vi "TBM HDI Wirebonds.vi"(6 "Match Offset (Pattern Matching 1)":cluster{"X":sgl, "Y":sgl}, 8 "Minimum Match Score (Pattern Matching 1)":sgl=600.0, 9 "controller in":refnum<k24>, 10 "Template for Encapsulation pattern matching":path, 11 "T/B/L/R":i32) -> (0 "error out":errorcluster, 1 "Number of Matches (Pattern Matching 1)":i32, 3 "Match(es) Found":bool)   [LabVIEW 2011]
uses:
  C:/Users/Admin/Desktop/Gantry Code Transfer/source/Code Transfer/Aerotech.A3200.dll
  Aerotech.A3200.dll
  Template change for pattern match.vi
  <vilib>/vision/driver/NI_Vision_Acquisition_Software.lvlib
  <vilib>/vision/NI_Vision_Development_Module.lvlib
panel:
  in  "Scale Factor":sgl=0.000429
  out "y rel move":dbl
  out "x rel move":dbl
  out "y":sgl
  out "x":sgl
  out "Image Out":T1(plugin-control)
  out "Calibrated Matches":T2(array[cluster]) {"Bounding Box"."y" format="%.2f"; "Bounding Box"."x" format="%.2f"; "Position"."y" format="%.2f"; "Position"."x" format="%.2f"; "Score" format="%.2f"; "Scale" format="%.2f"; "Angle" format="%.2f"}
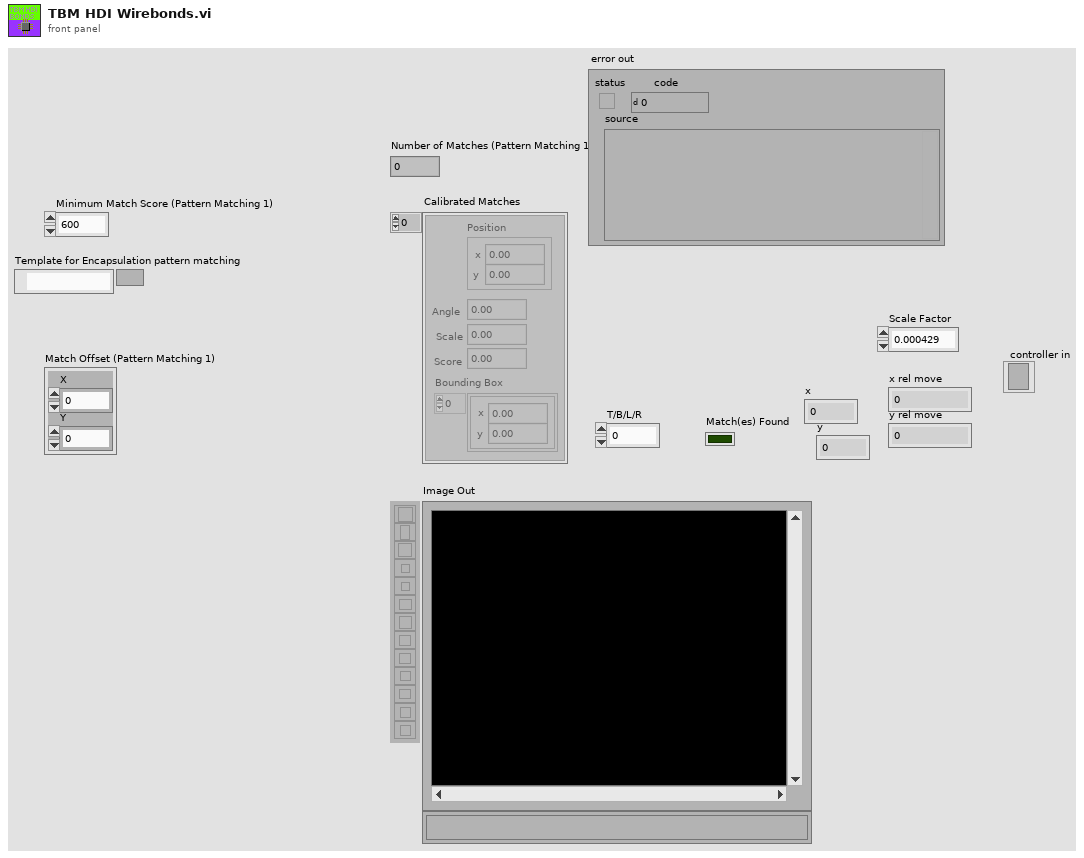
[diagram p1: front panel]
types:
  T1 = typedef "IMAQ Image.ctl" = refnum<image>
  T2 = cluster{"Position":cluster{"x":sgl, "y":sgl}, "Angle":sgl, "Scale":sgl, "Score":sgl, "Bounding Box":cluster{"x":sgl, "y":sgl}[]}[]
  T3 = cluster{"Global Rectangle":i32[], "Contours":cluster{"ID":enum32{"External", "Internal"}, "Type":u32, "Coordinates":i32[]}[]}
  T4 = typedef "IMAQdx.ctl" = refnum<k21>
  T5 = cluster{"Match Mode":u16, "Subpixel Accuracy":bool, "Rotation Angle Ranges (degrees) (Pattern Matching 1)":cluster{sgl, sgl}[]}
  T6 = cluster{"Global Rectangle":i32[], "Number of Matches Requested (Pattern Matching 1)":i32, "Minimum Match Score (Pattern Matching 1)":sgl}
  T7 = cluster{"Position":cluster{"x":sgl, "y":sgl}, "Angle":sgl, "Scale":sgl, "Score":sgl, "Bounding Box":cluster{"x":sgl, "y":sgl}[]}
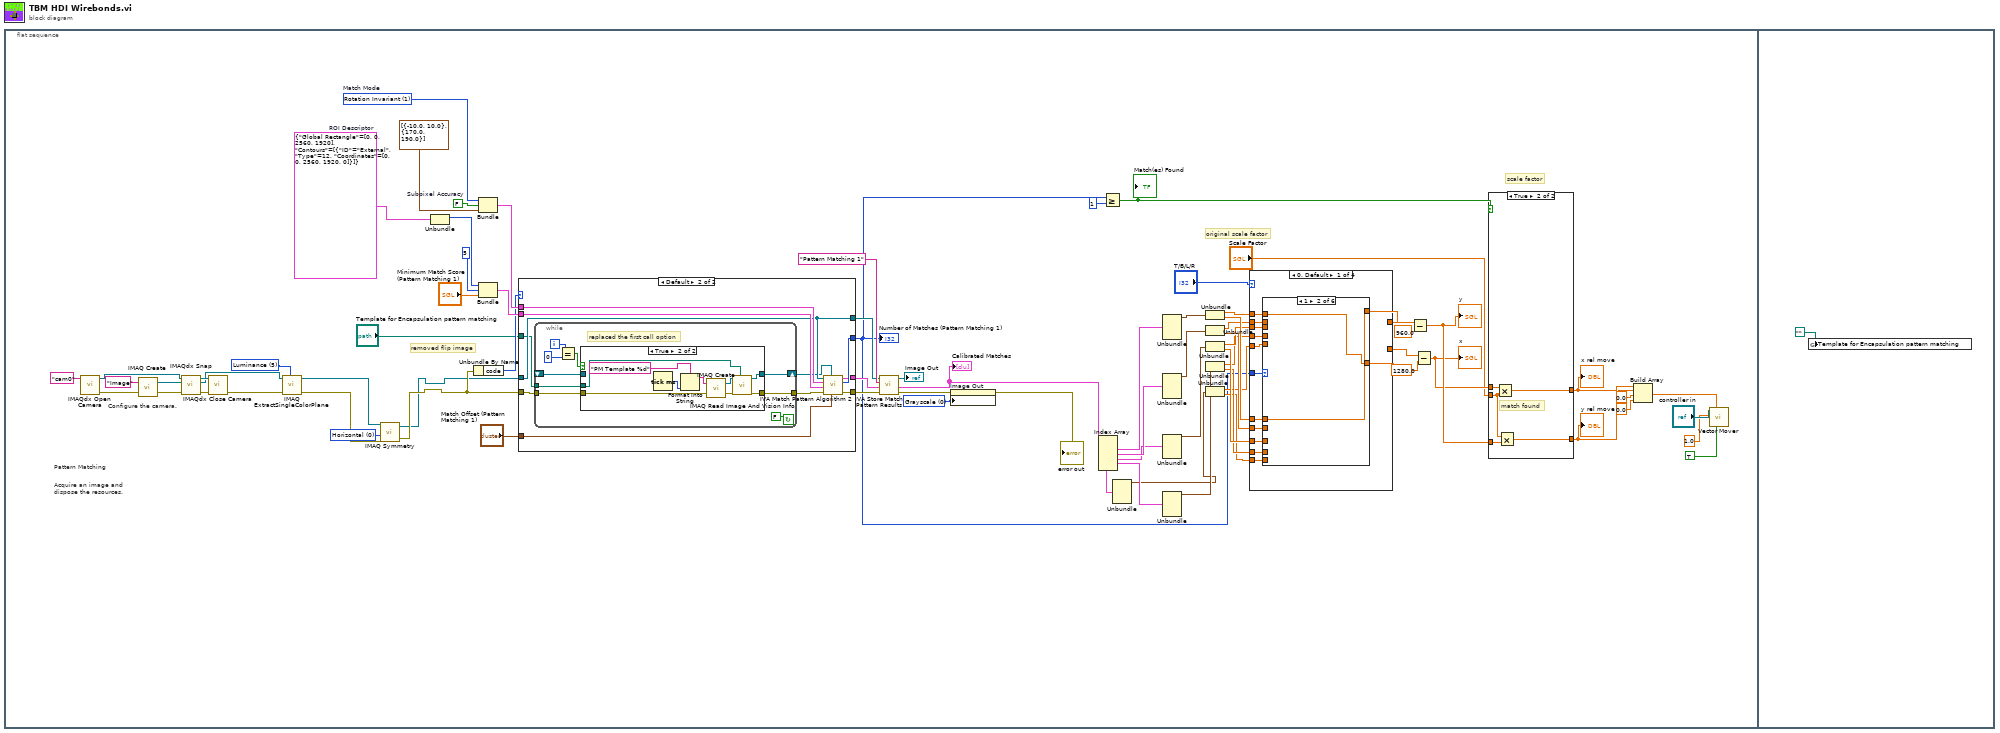
[diagram p0: block diagram]
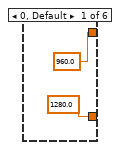
[diagram p2: hidden frame]
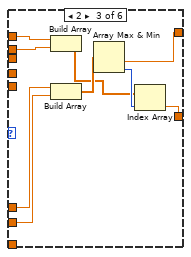
[diagram p3: hidden frame]
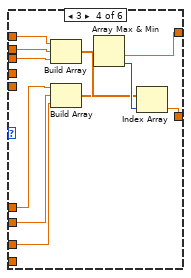
[diagram p4: hidden frame]
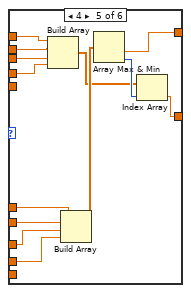
[diagram p5: hidden frame]
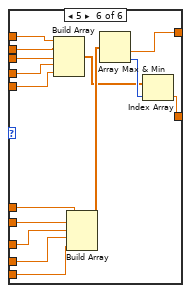
[diagram p6: hidden frame]
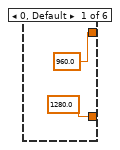
[diagram p8: hidden frame]
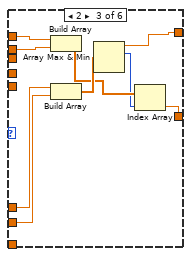
[diagram p9: hidden frame]
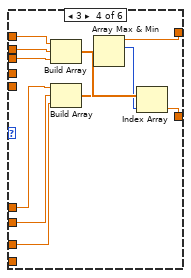
[diagram p10: hidden frame]
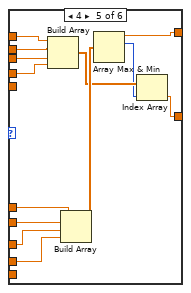
[diagram p11: hidden frame]
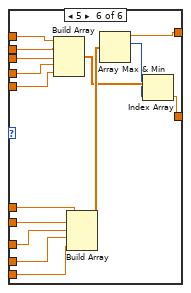
[diagram p12: hidden frame]
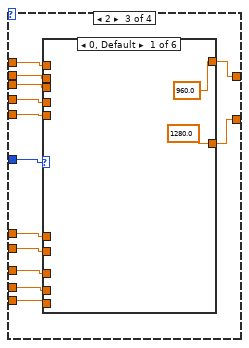
[diagram p13: hidden frame]
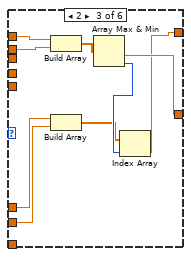
[diagram p15: hidden frame]
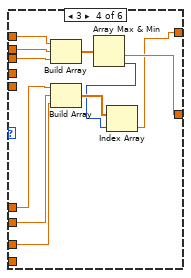
[diagram p16: hidden frame]
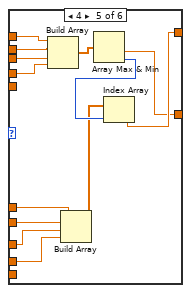
[diagram p17: hidden frame]
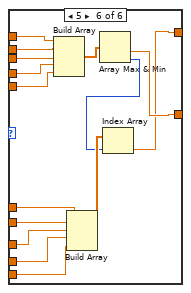
[diagram p18: hidden frame]
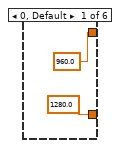
[diagram p20: hidden frame]
diagram:
  n1 = flat-sequence {
    frame #0 {
      w5 = u32 0 items=["Horizontal", "Vertical", "Central", "1st Diagonal", "2nd Diagonal"] ("Type of Symmetry")
      w47 = u32 0 items=["Grayscale", "Binary", "Gradient", "Rainbow", "Temperature", "User Defined"] ("Palette")
      w63 = FALSE  # Subpixel Accuracy
      w64 = u16 1 items=["Shift Invariant", "Rotation Invariant"]  # Match Mode
      w53 = T3 {"Global Rectangle"=[0, 0, 2560, 1920], "Contours"=[{"ID"=enum."External", "Type"=12, "Coordinates"=[0, 0, 2560, 1920, 0]}]}  # ROI Descriptor
      w66 = 5 items=["Red", "Green", "Blue", "Hue", "Saturation", "Luminance", "Value", "Intensity"] ("Color Plane")
      # "removed flip image"
      # "original scale factor"
      # "scale factor"
      # "Pattern Matching"
      # "Acquire an image and\ndispose the resources."
      # "Configure the camera."
      n2 = call <vilib>:"IMAQdx Open Camera.vi"("Session In"="cam0" ("Interface Name")) -> ("error out"=w73:errorcluster, "Session Out"=w67:T4)  [unwired: 9 in]
      n3 = call "IMAQ Create"("Image Name"="Image", "error in (no error)"=w73) -> ("New Image"=w69:T1, "error out"=w68:errorcluster)  [unwired: 3 in]
      n4 = call <vilib>:"IMAQdx Snap.vi"("error in"=w68, "Image In"=w69, "Session In"=w67) -> ("error out"=w71:errorcluster, "Image Out"=w65:T1, "Session Out"=w72:T4)  [unwired: 6 in]
      n5 = call <vilib>:"IMAQdx Close Camera.vi"("error in"=w71, "Session In"=w72) -> ("error out"=w70:errorcluster)  [unwired: 9 in]
      n6 = call "IMAQ ExtractSingleColorPlane"("Color Plane"=w66, "error in (no error)"=w70, "Image Src"=w65) -> ("error out"=w3:errorcluster, "Image Dst Out"=w4:T1)  [unwired: 7 in]
      n7 = call "IMAQ Symmetry"("error in (no error)"=w3, "Type of Symmetry"=w5, "Image Src"=w4) -> ("error out"=w2:errorcluster, "Image Dst Out"=w1:T1)  [unwired: 2 in]
      n8 = Unbundle(w53) -> ("Global Rectangle"=w52:i32[])  [unwired: 1 out]
      n9 = Unbundle By Name(w2) -> ("code"=w49:i32)
      n10 = Bundle("Match Mode"=w64, "Subpixel Accuracy"=w63, "Rotation Angle Ranges (degrees) (Pattern Matching 1)"=cluster{sgl, sgl}[] [{-10.0, 10.0}, {170.0, 190.0}]) -> (w61:T5)  [unwired: 1 in]
      n11 = Bundle("Global Rectangle"=w52, "Number of Matches Requested (Pattern Matching 1)"=5, "Minimum Match Score (Pattern Matching 1)"="Minimum Match Score (Pattern Matching 1)") -> (w58:T6)  [unwired: 1 in]
      n12 = case shown="Default" w49 {
        tunnel: "Template for Encapsulation pattern matching" -> [_ w346]
        tunnel: w2 -> [_ w345]
        tunnel: [_ w353] -> w7
        tunnel: w61 -> [_ w352]
        tunnel: w58 -> [_ w351]
        tunnel: "Match Offset (Pattern Matching 1)" -> [_ w350]
        tunnel: w1 -> [w342 w347]
        tunnel: [_ w349] -> w55
        tunnel: [_ w348] -> w51
        tunnel: [w342 w347] -> w50
        frame -1074396199, -1074396198 {
          # "Discard\nCoordinate\nSystem Error"
        }
        frame Default {
          n13 = while {
            shift-right: [w362] -> w343
            shift-left: _ -> [w361]
            tunnel: [w359] -> w344
            tunnel: w345 -> [w358]
            tunnel: w346 -> [w357]
            i -> [w356]
            stop <- FALSE continue-if-true
            # "replaced the first call option"
            n14 = Equal?(x=w356, y=0) -> (x = y?=w354:bool)
            n15 = case shown="True" w354 {
              tunnel: [w364 w370] -> w362
              tunnel: w361 -> [w364 _]
              tunnel: [w363 w367] -> w359
              tunnel: w358 -> [w363 w366]
              tunnel: w357 -> [_ w365]
              frame False {
              }
              frame True {
                n16 = Tick Count (ms)() -> (millisecond timer value=w373:u32)
                n17 = Format Into String(format string="PM Template %d" ("Image Name"), w373) -> (resulting string=w372:string)  [unwired: 2 in, 1 out]
                n18 = call "IMAQ Create"("Image Name"=w372, "error in (no error)"=w366) -> ("New Image"=w369:T1, "error out"=w368:errorcluster)  [unwired: 3 in]
                n19 = call "IMAQ Read Image And Vision Info"("File Path"=w365, "error in (no error)"=w368, "Image"=w369) -> ("error out"=w367:errorcluster, "Image Out"=w370:T1)  [unwired: 6 in, 1 out]
              }
            }
          }
          n20 = call <vilib>:"IVA Match Pattern Algorithm 2.vi"("Match Offset"=w350, "Image Template"=w343, "error in (no error)"=w344, "Match Parameters"=w351, "Setup Match Parameters"=w352, "Image"=w347) -> ("error out"=w349:errorcluster, "Number of Matches"=w353:i32, "Matches"=w348:T2)  [unwired: 3 in]
        }
      }
      "Number of Matches (Pattern Matching 1)" <- w7
      n21 = call <vilib>:"IVA Store Match Pattern Results.vi"("error in (no error)"=w55, "Matches"=w51, "Step Name"="Pattern Matching 1", "Image in"=w50) -> ("error out"=w54:errorcluster, "Calibrated Matches"=w8:T2, "Image dup"=→"Image Out":T1)  [unwired: 5 in]
      "Calibrated Matches" <- w8
      "error out" <- w54
      n22 = property on="Image Out" class="ImageControl"(error in=w54, "Palette:Palette Type"=w47) -> ()  [unwired: 1 in, 2 out]
      n23 = Index Array(array=w8) -> (element #1=w43:T7, element #2=w42:T7, element #3=w41:T7, element #4=w40:T7, element #5=w20:T7)  [unwired: 5 in]
      n24 = Greater Or Equal?(x=w7, y=1) -> (x >= y?=w33:bool)
      "Match(es) Found" <- w33
      n25 = Unbundle(w20) -> ("Position"=w19:cluster{"x":sgl, "y":sgl})  [unwired: 4 out]
      n26 = Unbundle(w43) -> ("Position"=w36:cluster{"x":sgl, "y":sgl})  [unwired: 4 out]
      n27 = Unbundle(w42) -> ("Position"=w37:cluster{"x":sgl, "y":sgl})  [unwired: 4 out]
      n28 = Unbundle(w41) -> ("Position"=w38:cluster{"x":sgl, "y":sgl})  [unwired: 4 out]
      n29 = Unbundle(w40) -> ("Position"=w39:cluster{"x":sgl, "y":sgl})  [unwired: 4 out]
      n30 = Unbundle(w36) -> ("x"=w30:sgl, "y"=w29:sgl)
      n31 = Unbundle(w37) -> ("x"=w28:sgl, "y"=w27:sgl)
      n32 = Unbundle(w38) -> ("x"=w25:sgl, "y"=w24:sgl)
      n33 = Unbundle(w39) -> ("x"=w21:sgl, "y"=w23:sgl)
      n34 = Unbundle(w19) -> ("x"=w18:sgl, "y"=w17:sgl)
      n35 = case shown="0, Default" "T/B/L/R" {
        tunnel: w30 -> [w88 w153 w218 w283]
        tunnel: w29 -> [w87 w148 w213 w278]
        tunnel: w28 -> [w86 w152 w217 w282]
        tunnel: w27 -> [w85 w147 w212 w277]
        tunnel: [w84 w141 w206 w271] -> w26
        tunnel: w25 -> [w83 w151 w216 w281]
        tunnel: w24 -> [w82 w146 w211 w276]
        tunnel: w23 -> [w81 w145 w210 w275]
        tunnel: [w80 w142 w207 w272] -> w22
        tunnel: w21 -> [w79 w150 w215 w280]
        tunnel: w18 -> [w78 w149 w214 w279]
        tunnel: w17 -> [w77 w144 w209 w274]
        tunnel: w7 -> [w76 w143 w208 w273]
        frame 0, Default {
          n36 = case shown="1" w76 {
            tunnel: w88 -> [_ w91 w101 w109 w122 w137]
            tunnel: w87 -> [_ w92 w99 w106 w118 w133]
            tunnel: [sgl 960.0 ("y") w92 w96 w111 w124 w139] -> w84
            tunnel: w86 -> [_ _ w100 w108 w121 w136]
            tunnel: w85 -> [_ _ w98 w105 w117 w132]
            tunnel: w83 -> [_ _ _ w107 w120 w135]
            tunnel: w82 -> [_ _ _ w104 w116 w131]
            tunnel: w81 -> [_ _ _ _ w115 w130]
            tunnel: [sgl 1280.0 ("x") w91 w93 w110 w123 w138] -> w80
            tunnel: w79 -> [_ _ _ _ w119 w134]
            tunnel: w78 -> [_ _ _ _ _ w127]
            tunnel: w77 -> [_ _ _ _ _ w126]
            frame 0, Default {
            }
            frame 1 {
            }
            frame 2 {
              n37 = Build Array(w101, w100) -> (w94:sgl[])
              n38 = Build Array(w99, w98) -> (w95:sgl[])
              n39 = Array Max & Min(array=w95) -> (min value=w96:sgl, min index (indices)=w97:i32)  [unwired: 2 out]
              n40 = Index Array(array=w94, index=w97) -> (element=w93:sgl)
            }
            frame 3 {
              n41 = Build Array(w109, w108, w107) -> (w103:sgl[])
              n42 = Build Array(w106, w105, w104) -> (w102:sgl[])
              n43 = Array Max & Min(array=w102) -> (min value=w111:sgl, min index (indices)=w112:i32)  [unwired: 2 out]
              n44 = Index Array(array=w103, index=w112) -> (element=w110:sgl)
            }
            frame 4 {
              n45 = Build Array(w122, w121, w120, w119) -> (w113:sgl[])
              n46 = Build Array(w118, w117, w116, w115) -> (w114:sgl[])
              n47 = Array Max & Min(array=w114) -> (min value=w124:sgl, min index (indices)=w125:i32)  [unwired: 2 out]
              n48 = Index Array(array=w113, index=w125) -> (element=w123:sgl)
            }
            frame 5 {
              n49 = Build Array(w137, w136, w135, w134, w127) -> (w128:sgl[])
              n50 = Build Array(w133, w132, w131, w130, w126) -> (w129:sgl[])
              n51 = Array Max & Min(array=w129) -> (min value=w139:sgl, min index (indices)=w140:i32)  [unwired: 2 out]
              n52 = Index Array(array=w128, index=w140) -> (element=w138:sgl)
            }
          }
        }
        frame 1 {
          n53 = case shown="1" w143 {
            tunnel: w153 -> [_ w156 w166 w176 w189 w204]
            tunnel: w148 -> [_ w157 w164 w173 w185 w200]
            tunnel: [sgl 960.0 ("y") w157 w158 w167 w178 w192] -> w141
            tunnel: w152 -> [_ _ w165 w175 w188 w203]
            tunnel: w147 -> [_ _ w163 w172 w184 w199]
            tunnel: w151 -> [_ _ _ w174 w187 w202]
            tunnel: w146 -> [_ _ _ w171 w183 w198]
            tunnel: w145 -> [_ _ _ _ w182 w197]
            tunnel: [sgl 1280.0 ("x") w156 w160 w177 w190 w205] -> w142
            tunnel: w150 -> [_ _ _ _ w186 w201]
            tunnel: w149 -> [_ _ _ _ _ w194]
            tunnel: w144 -> [_ _ _ _ _ w193]
            frame 0, Default {
            }
            frame 1 {
            }
            frame 2 {
              n54 = Build Array(w166, w165) -> (w161:sgl[])
              n55 = Build Array(w164, w163) -> (w162:sgl[])
              n56 = Array Max & Min(array=w162) -> (max value=w158:sgl, max index (indices)=w159:i32)  [unwired: 2 out]
              n57 = Index Array(array=w161, index=w159) -> (element=w160:sgl)
            }
            frame 3 {
              n58 = Build Array(w176, w175, w174) -> (w170:sgl[])
              n59 = Build Array(w173, w172, w171) -> (w169:sgl[])
              n60 = Array Max & Min(array=w169) -> (max value=w167:sgl, max index (indices)=w168:i32)  [unwired: 2 out]
              n61 = Index Array(array=w170, index=w168) -> (element=w177:sgl)
            }
            frame 4 {
              n62 = Build Array(w189, w188, w187, w186) -> (w180:sgl[])
              n63 = Build Array(w185, w184, w183, w182) -> (w181:sgl[])
              n64 = Array Max & Min(array=w181) -> (max value=w178:sgl, max index (indices)=w179:i32)  [unwired: 2 out]
              n65 = Index Array(array=w180, index=w179) -> (element=w190:sgl)
            }
            frame 5 {
              n66 = Build Array(w204, w203, w202, w201, w194) -> (w195:sgl[])
              n67 = Build Array(w200, w199, w198, w197, w193) -> (w196:sgl[])
              n68 = Array Max & Min(array=w196) -> (max value=w192:sgl, max index (indices)=w191:i32)  [unwired: 2 out]
              n69 = Index Array(array=w195, index=w191) -> (element=w205:sgl)
            }
          }
        }
        frame 2 {
          n70 = case shown="0, Default" w208 {
            tunnel: w218 -> [_ w221 w231 w242 w254 w270]
            tunnel: w213 -> [_ w222 w229 w239 w250 w266]
            tunnel: [sgl 960.0 ("y") w222 w223 w232 w244 w256] -> w206
            tunnel: w217 -> [_ _ w230 w241 w253 w269]
            tunnel: w212 -> [_ _ w228 w238 w249 w265]
            tunnel: w216 -> [_ _ _ w240 w252 w268]
            tunnel: w211 -> [_ _ _ w237 w248 w264]
            tunnel: w210 -> [_ _ _ _ w247 w263]
            tunnel: [sgl 1280.0 ("x") w221 w226 w233 w243 w257] -> w207
            tunnel: w215 -> [_ _ _ _ w251 w267]
            tunnel: w214 -> [_ _ _ _ _ w262]
            tunnel: w209 -> [_ _ _ _ _ w261]
            frame 0, Default {
            }
            frame 1 {
            }
            frame 2 {
              n71 = Build Array(w231, w230) -> (w227:sgl[])
              n72 = Build Array(w229, w228) -> (w224:sgl[])
              n73 = Array Max & Min(array=w227) -> (min value=w226:sgl, min index (indices)=w225:i32)  [unwired: 2 out]
              n74 = Index Array(array=w224, index=w225) -> (element=w223:sgl)
            }
            frame 3 {
              n75 = Build Array(w242, w241, w240) -> (w236:sgl[])
              n76 = Build Array(w239, w238, w237) -> (w235:sgl[])
              n77 = Array Max & Min(array=w236) -> (min value=w233:sgl, min index (indices)=w234:i32)  [unwired: 2 out]
              n78 = Index Array(array=w235, index=w234) -> (element=w232:sgl)
            }
            frame 4 {
              n79 = Build Array(w254, w253, w252, w251) -> (w245:sgl[])
              n80 = Build Array(w250, w249, w248, w247) -> (w246:sgl[])
              n81 = Array Max & Min(array=w245) -> (min value=w243:sgl, min index (indices)=w255:i32)  [unwired: 2 out]
              n82 = Index Array(array=w246, index=w255) -> (element=w244:sgl)
            }
            frame 5 {
              n83 = Build Array(w270, w269, w268, w267, w262) -> (w258:sgl[])
              n84 = Build Array(w266, w265, w264, w263, w261) -> (w260:sgl[])
              n85 = Array Max & Min(array=w258) -> (min value=w257:sgl, min index (indices)=w259:i32)  [unwired: 2 out]
              n86 = Index Array(array=w260, index=w259) -> (element=w256:sgl)
            }
          }
        }
        frame 3 {
          n87 = case shown="1" w273 {
            tunnel: w283 -> [_ w286 w296 w307 w320 w335]
            tunnel: w278 -> [_ w287 w294 w304 w316 w331]
            tunnel: [sgl 960.0 ("y") w287 w290 w299 w310 w323] -> w271
            tunnel: w282 -> [_ _ w295 w306 w319 w334]
            tunnel: w277 -> [_ _ w293 w303 w315 w330]
            tunnel: w281 -> [_ _ _ w305 w318 w333]
            tunnel: w276 -> [_ _ _ w302 w314 w329]
            tunnel: w275 -> [_ _ _ _ w313 w328]
            tunnel: [sgl 1280.0 ("x") w286 w289 w298 w309 w322] -> w272
            tunnel: w280 -> [_ _ _ _ w317 w332]
            tunnel: w279 -> [_ _ _ _ _ w327]
            tunnel: w274 -> [_ _ _ _ _ w326]
            frame 0, Default {
            }
            frame 1 {
            }
            frame 2 {
              n88 = Build Array(w296, w295) -> (w292:sgl[])
              n89 = Build Array(w294, w293) -> (w291:sgl[])
              n90 = Array Max & Min(array=w292) -> (max value=w289:sgl, max index (indices)=w288:i32)  [unwired: 2 out]
              n91 = Index Array(array=w291, index=w288) -> (element=w290:sgl)
            }
            frame 3 {
              n92 = Build Array(w307, w306, w305) -> (w301:sgl[])
              n93 = Build Array(w304, w303, w302) -> (w300:sgl[])
              n94 = Array Max & Min(array=w301) -> (max value=w298:sgl, max index (indices)=w297:i32)  [unwired: 2 out]
              n95 = Index Array(array=w300, index=w297) -> (element=w299:sgl)
            }
            frame 4 {
              n96 = Build Array(w320, w319, w318, w317) -> (w311:sgl[])
              n97 = Build Array(w316, w315, w314, w313) -> (w312:sgl[])
              n98 = Array Max & Min(array=w311) -> (max value=w309:sgl, max index (indices)=w308:i32)  [unwired: 2 out]
              n99 = Index Array(array=w312, index=w308) -> (element=w310:sgl)
            }
            frame 5 {
              n100 = Build Array(w335, w334, w333, w332, w327) -> (w324:sgl[])
              n101 = Build Array(w331, w330, w329, w328, w326) -> (w325:sgl[])
              n102 = Array Max & Min(array=w324) -> (max value=w322:sgl, max index (indices)=w321:i32)  [unwired: 2 out]
              n103 = Index Array(array=w325, index=w321) -> (element=w323:sgl)
            }
          }
        }
      }
      n104 = Subtract(x=w26, y=sgl 960.0) -> (x-y=w46:sgl)
      "y" <- w46
      n105 = Subtract(x=w22, y=sgl 1280.0) -> (x-y=w45:sgl)
      "x" <- w45
      n106 = case shown="True" w33 {
        tunnel: w46 -> [_ w341]
        tunnel: w45 -> [_ w340]
        tunnel: [w336 w339] -> w31
        tunnel: [w336 w338] -> w32
        tunnel: "Scale Factor" -> [_ w337]
        frame False {
          w336 = sgl 0.0
          # "no match found"
        }
        frame True {
          # "match found"
          n107 = Multiply(x=w340, y=w337) -> (x*y=w339:sgl)
          n108 = Multiply(x=w337, y=w341) -> (x*y=w338:sgl)
        }
      }
      "x rel move" <- w31
      "y rel move" <- w32
      n109 = Build Array(w32, w31, 0.0 ("element"), 0.0 ("element")) -> (w9:dbl[])
      n110 = call "Vector Mover.vi"("Absolute/Relative (F/T)"=TRUE, "Movement Vector"=w9, "Vector Speed"=1.0, "controller in"="controller in") -> ()  [unwired: 2 in, 4 out]
    }
    frame #1 {
      n111 = global write "Template change for pattern match.vi" "Template for Encapsulation pattern matching"(path "") -> ()
    }
  }
